vi "RAHHH TEST.vi"() -> ()   [LabVIEW 2009]
uses:
  <vilib>/LabVIEW Targets/FPGA/cRIO/shared/nicrio_ModuleControls/nicrio_cRIO-9871_BaudRateEnum.ctl
  <vilib>/LabVIEW Targets/FPGA/cRIO/shared/nicrio_ModuleControls/nicrio_cRIO-9871_DataBitsEnum.ctl
  <vilib>/LabVIEW Targets/FPGA/cRIO/shared/nicrio_ModuleControls/nicrio_cRIO-9871_StopBitsEnum.ctl
  <vilib>/LabVIEW Targets/FPGA/cRIO/shared/nicrio_ModuleControls/nicrio_cRIO-9871_ParityEnum.ctl
  <vilib>/LabVIEW Targets/FPGA/cRIO/shared/nicrio_ModuleControls/nicrio_cRIO-9871_FlowControlEnum.ctl
  <vilib>/userDefined/High Color/nirio_resource_hc.ctl
  <vilib>/rvi/interface/nirviOpenFPGA/nirviOpenFPGA.xnode
  FPGA Bitfiles/Q_IGVC_2010.lvproj_FPGA Target_GPS diagnostic.vi.lvbitx
  <vilib>/FPGAPlugInAG/cRIO-9113/nirviIntfOpen_cRIO-9113.vi
  <vilib>/rvi/interface/nirviCloseFPGA/nirviCloseFPGA.xnode
  <vilib>/FPGAPlugInAG/cRIO-9113/nirviIntfClose_cRIO-9113.vi
  SS FPGA VI Ref.ctl
panel:
  in  "String":string
  out "concatenated string":string
  in  "stop":bool
  in  "Flow Control 4":T1
  in  "Parity 4":T2
  in  "Stop Bits 4":T3
  in  "Data Bits 4":T4=enum."8"
  in  "Baud Rate 4":T5=enum."4800 bps"
  in  "Flow Control 3":T1
  in  "Parity 3":T2
  in  "Stop Bits 3":T3
  in  "Data Bits 3":T4=enum."8"
  in  "Baud Rate 3":T5=enum."4800 bps"
  in  "Flow Control 2":T1
  in  "Parity 2":T2
  in  "Stop Bits 2":T3
  in  "Data Bits 2":T4=enum."8"
  in  "Baud Rate 2":T5=enum."4800 bps"
  in  "Flow Control":T1
  in  "Parity":T2
  in  "Stop Bits":T3
  in  "Data Bits":T4=enum."8"
  in  "Baud Rate":T5=enum."19.2 kbps"
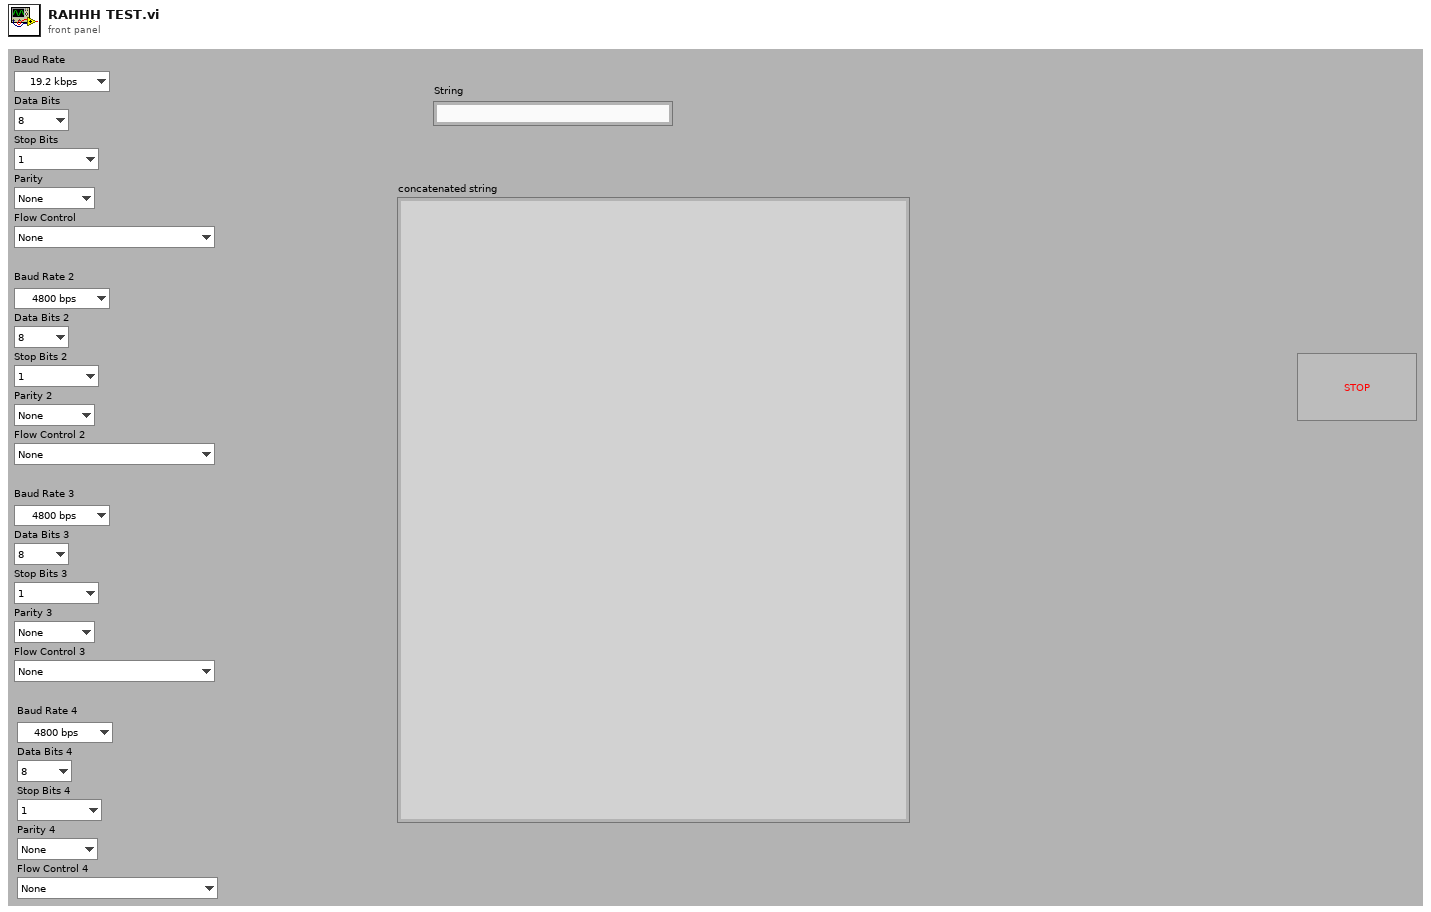
[diagram p1: front panel]
types:
  T1 = typedef "nicrio_cRIO-9871_FlowControlEnum.ctl" = enum8{"None", "Software (XON / XOFF)", "Hardware (RTS / CTS)"}
  T2 = typedef "nicrio_cRIO-9871_ParityEnum.ctl" = enum8{"None", "Odd", "Even", "Mark", "Space"}
  T3 = typedef "nicrio_cRIO-9871_StopBitsEnum.ctl" = enum8{"1", "1.5", "2"}
  T4 = typedef "nicrio_cRIO-9871_DataBitsEnum.ctl" = enum8{"5", "6", "7", "8"}
  T5 = typedef "nicrio_cRIO-9871_BaudRateEnum.ctl" = enum16{"75 bps", "110 bps", "134 bps", "150 bps", "300 bps", "600 bps", "1200 bps", "1800 bps", "2400 bps", "4800 bps", "7200 bps", "9600 bps", "14.4 kbps", "19.2 kbps", "28.8 kbps", "38.4 kbps", "57.6 kbps", "115.2 kbps", "230.4 kbps", "460.8 kbps", "921.6 kbps"}
  T6 = typedef "nirio_resource_hc.ctl" = tag
  T7 = typedef "SS FPGA VI Ref.ctl" = refnum<k20>
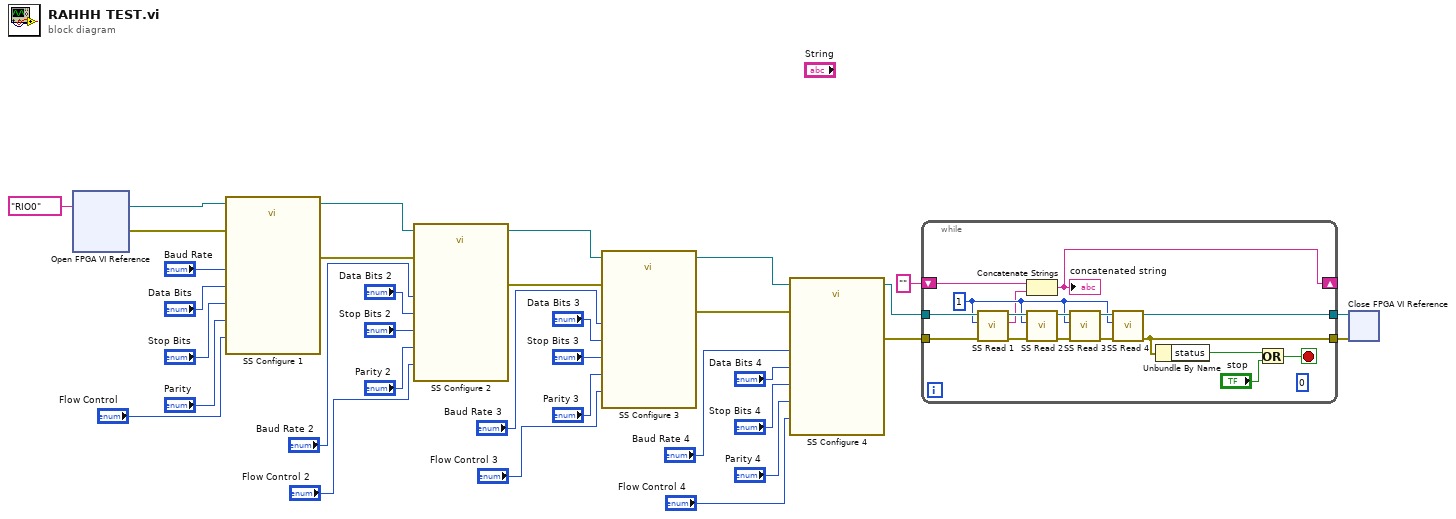
[diagram p0: block diagram]
diagram:
  n1 = xnode "Open FPGA VI Reference"("resource name"=T6 "RIO0") -> ("FPGA VI Reference Out"=w27:refnum<k20>, "error out"=w28:errorcluster)  [unwired: 1 in]
  n2 = call "SS Configure 1.vi"("Flow Control"="Flow Control", "Parity"="Parity", "Stop Bits"="Stop Bits", "error in (no error)"=w28, "Data Bits"="Data Bits", "Baud Rate"="Baud Rate", "Simple Serial Ref in"=w27) -> ("error out"=w34:errorcluster, "Simple Serial Ref out"=w33:T7)  [unwired: 3 in]
  n3 = call "SS Configure 2.vi"("Flow Control"="Flow Control 2", "Parity"="Parity 2", "Stop Bits"="Stop Bits 2", "error in (no error)"=w34, "Data Bits"="Data Bits 2", "Baud Rate"="Baud Rate 2", "Simple Serial Ref in"=w33) -> ("error out"=w32:errorcluster, "Simple Serial Ref out"=w31:T7)  [unwired: 3 in]
  n4 = call "SS Configure 3.vi"("Flow Control"="Flow Control 3", "Parity"="Parity 3", "Stop Bits"="Stop Bits 3", "error in (no error)"=w32, "Data Bits"="Data Bits 3", "Baud Rate"="Baud Rate 3", "Simple Serial Ref in"=w31) -> ("error out"=w30:errorcluster, "Simple Serial Ref out"=w29:T7)  [unwired: 3 in]
  n5 = call "SS Configure 4.vi"("Flow Control"="Flow Control 4", "Parity"="Parity 4", "Stop Bits"="Stop Bits 4", "error in (no error)"=w30, "Data Bits"="Data Bits 4", "Baud Rate"="Baud Rate 4", "Simple Serial Ref in"=w29) -> ("error out"=w5:errorcluster, "Simple Serial Ref out"=w4:T7)  [unwired: 3 in]
  n6 = while {
    tunnel: w5 -> [w47]
    tunnel: w4 -> [w51]
    tunnel: [w40] -> w3
    tunnel: [w38] -> w2
    shift-right: [w35] -> _
    shift-left: "" ("Data") -> [w37]
    stop <- w41 stop-if-true
    (unwired) 0 ("index")
    w46 = 1 ("Number of Bytes to Read")
    n7 = call "SS Read 1.vi"("error in (no error)"=w47, "Number of Bytes to Read"=w46, "FPGA VI Reference in"=w51) -> ("error out"=w45:errorcluster, "Data"=w36:string, "FPGA VI Reference out"=w50:T7)  [unwired: 6 in]
    n8 = Concatenate Strings(w37, w36) -> (w35:string)
    "concatenated string" <- w35
    n9 = call "SS Read 2.vi"("error in (no error)"=w45, "Number of Bytes to Read"=w46, "FPGA VI Reference in"=w50) -> ("error out"=w44:errorcluster, "FPGA VI Reference out"=w49:T7)  [unwired: 6 in, 1 out]
    n10 = call "SS Read 3.vi"("error in (no error)"=w44, "Number of Bytes to Read"=w46, "FPGA VI Reference in"=w49) -> ("error out"=w43:errorcluster, "FPGA VI Reference out"=w48:T7)  [unwired: 6 in, 1 out]
    n11 = call "SS Read 4.vi"("error in (no error)"=w43, "Number of Bytes to Read"=w46, "FPGA VI Reference in"=w48) -> ("error out"=w40:errorcluster, "FPGA VI Reference out"=w38:T7)  [unwired: 6 in, 1 out]
    n12 = Unbundle By Name(w40) -> ("status"=w39:bool)
    n13 = Or(x=w39, y="stop") -> (x .or. y?=w41:bool)
  }
  n14 = xnode "Close FPGA VI Reference"("FPGA VI Reference In"=w2, "error in"=w3) -> ()  [unwired: 1 out]
